vi "timestamp_dategmt.vi"(1 "time stamp":timestamp) -> (0 "String":string)   [LabVIEW 2011]
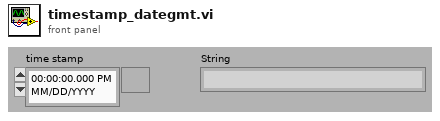
[diagram p1: front panel]
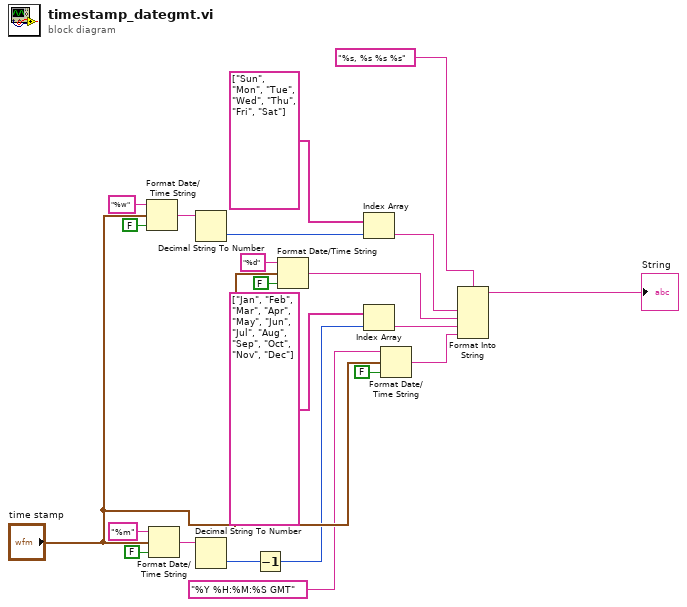
[diagram p0: block diagram]
diagram:
  n1 = Format Date/Time String(time format string (%c)="%w", seconds (now)="time stamp", UTC format=FALSE) -> (date/time string=w13:string)
  n2 = Format Date/Time String(time format string (%c)="%m", seconds (now)="time stamp", UTC format=FALSE) -> (date/time string=w9:string)
  n3 = Decimal String To Number(string=w13) -> (number=w1:i32)  [unwired: 2 in, 1 out]
  n4 = Decimal String To Number(string=w9) -> (number=w11:i32)  [unwired: 2 in, 1 out]
  n5 = Decrement(x=w11) -> (x-1=w12:i32)
  n6 = Format Date/Time String(time format string (%c)="%d", seconds (now)="time stamp", UTC format=FALSE) -> (date/time string=w19:string)
  n7 = Index Array(array=string[] ["Sun", "Mon", "Tue", "Wed", "Thu", "Fri", "Sat"], index=w1) -> (element=w2:string)
  n8 = Index Array(array=string[] ["Jan", "Feb", "Mar", "Apr", "May", "Jun", "Jul", "Aug", "Sep", "Oct", "Nov", "Dec"], index=w12) -> (element=w16:string)
  n9 = Format Date/Time String(time format string (%c)="%Y %H:%M:%S GMT", seconds (now)="time stamp", UTC format=FALSE) -> (date/time string=w17:string)
  n10 = Format Into String(format string="%s, %s %s %s", w2, w19, w16, w17) -> (resulting string=→"String":string)  [unwired: 2 in, 1 out]
